vi "624WPI_CameraSend Image String To PC 1.0.0.0.vi"(8 "error in (no error)":errorcluster, 10 "String":string, 11 "TCP Connection ID":refnum<k5>) -> (0 "error out":errorcluster, 3 "TCP Connection ID out":refnum<k5>)   [LabVIEW 2014]
doc: "Version 1.0.0.0 of the image transfer protocol.\n\nSend the version information first and then sends a raw JPEG string to the PC.\n\nThis software is licensed. Open the labview\\readme\\WPI Robotics Library Open Source License.txt file for more information."
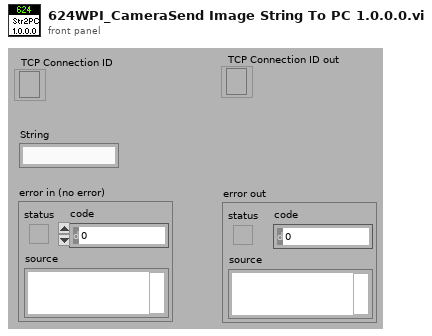
[diagram p1: front panel]
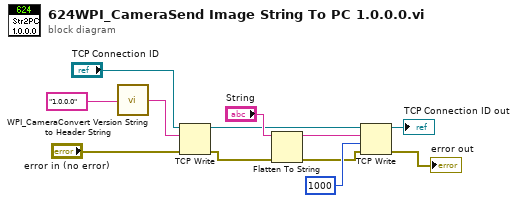
[diagram p0: block diagram]
diagram:
  n1 = call <vilib>:"WPI_CameraConvert Version String to Header String.vi"("String"="1.0.0.0") -> ("string"=w6:string)  [unwired: 14 out]
  n2 = TCP Write(connection ID="TCP Connection ID", data in=w6, error in (no error)="error in (no error)") -> (connection ID out=w4:refnum<k5>, error out=w2:errorcluster)  [unwired: 2 out]
  n3 = Flatten To String(anything="String", error in (no error)=w2) -> (data string=w9:string, error out=w8:errorcluster)  [unwired: 3 out]
  n4 = TCP Write(connection ID=w4, data in=w9, error in (no error)=w8, 9:1000 ("timeout ms (25000)")) -> (connection ID out=→"TCP Connection ID out":refnum<k5>, error out=→"error out":errorcluster)  [unwired: 1 out]
